vi "_TEST_ObjCacher.vi"() -> ()   [LabVIEW 2017]
uses:
  ObjectCacher-Operation.ctl
  a46cdb9f-ccaa-43c4-a046-aebf299bd719.vi
  e83d7f05-6254-462c-8cdd-b9405a50ceee.vi
  770d1e0a-3b1e-40e7-88fb-791e80b0e344.vi
  a343c373-1cd9-49a8-b7bb-35b9f087bed4.vi
  <vilib>/Utility/error.llb/Clear Errors.vi
  <userlib>/_OpenG.lib/md5/md5.llb/MD5 Message Digest (Hexadecimal String)__ogtk.vi
panel:
  out "names":string[](array[string])
  out "element 3":string
  out "data string 3":string
  out "element 2":string
  out "data string 2":string
  out "data string":string
  out "element":string
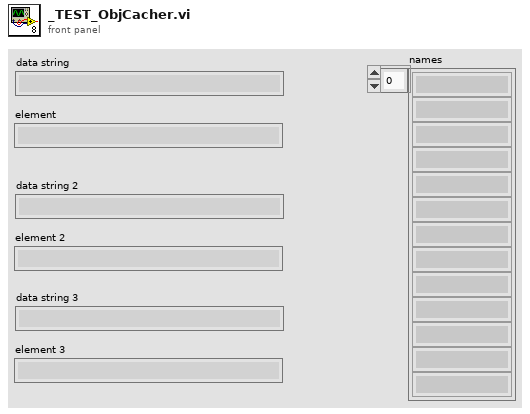
[diagram p1: front panel]
types:
  T1 = typedef "ObjectCacher-Operation.ctl" = enum16{"Reset", "Set", "Get", "Delete", "List", "<NONE>"}
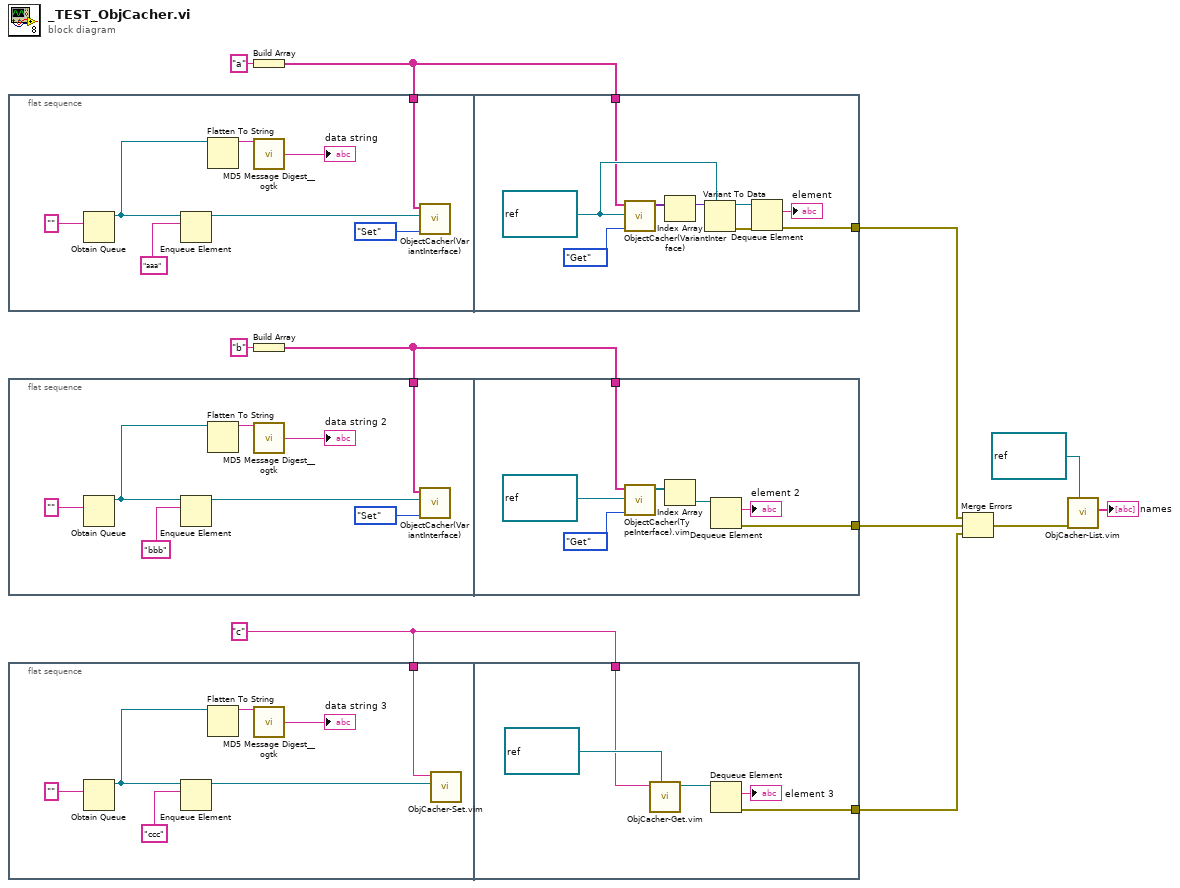
[diagram p0: block diagram]
diagram:
  w7 = "c" ("key")
  n1 = flat-sequence {
    tunnel: w10 -> [w12]
    tunnel: w10 -> [w24]
    tunnel: [w20] -> w4
    frame #0 {
      n2 = Obtain Queue(element data type="") -> (queue out=w16:refnum<queue>)  [unwired: 4 in, 2 out]
      n3 = Enqueue Element(queue=w16, element="aaa") -> (queue out=w18:refnum<queue>)  [unwired: 2 in, 2 out]
      n4 = Flatten To String(anything=w16) -> (data string=w15:string)  [unwired: 3 in, 2 out]
      n5 = call-poly <userlib>:"MD5 Message Digest__ogtk.vi"("Message"=w15) -> ("MD5 Message Digest"=→"data string":string)
      n6 = call "ObjectCacher(VariantInterface).vi"("Enum(Get)"=ObjectCacher-Operation."Set", "Variant"=w18, "key"=w12) -> ()  [unwired: 5 in, 4 out]
    }
    frame #1 {
      w28 = refnum<queue> refnum ("queue out")
      n7 = call "ObjectCacher(VariantInterface).vi"("Enum(Get)"=ObjectCacher-Operation."Get", "Variant"=w28, "key"=w24) -> ("values"=w22:variant[])  [unwired: 5 in, 3 out]
      n8 = Index Array(array=w22) -> (element=w21:variant)  [unwired: 1 in]
      n9 = Variant To Data(type=w28, Variant=w21) -> (data=w27:refnum<queue>, error out=w26:errorcluster)  [unwired: 1 in]
      n10 = Dequeue Element(queue=w27, error in (no error)=w26) -> (element=→"element":string, error out=w20:errorcluster)  [unwired: 1 in, 2 out]
    }
  }
  n11 = flat-sequence {
    tunnel: w9 -> [w29]
    tunnel: w9 -> [w41]
    tunnel: [w37] -> w6
    frame #0 {
      n12 = Obtain Queue(element data type="") -> (queue out=w33:refnum<queue>)  [unwired: 4 in, 2 out]
      n13 = Enqueue Element(queue=w33, element="bbb") -> (queue out=w35:refnum<queue>)  [unwired: 2 in, 2 out]
      n14 = Flatten To String(anything=w33) -> (data string=w32:string)  [unwired: 3 in, 2 out]
      n15 = call-poly <userlib>:"MD5 Message Digest__ogtk.vi"("Message"=w32) -> ("MD5 Message Digest"=→"data string 2":string)
      n16 = call "ObjectCacher(VariantInterface).vi"("Enum(Get)"=ObjectCacher-Operation."Set", "Variant"=w35, "key"=w29) -> ()  [unwired: 5 in, 4 out]
    }
    frame #1 {
      n17 = call "ObjectCacher(TypeInterface).vim"("Enum(Get)"=ObjectCacher-Operation."Get", "Variant"=refnum<queue> refnum ("queue out"), "key"=w41) -> ("values"=w39:refnum<queue>[])  [unwired: 5 in, 3 out]
      n18 = Index Array(array=w39) -> (element=w38:refnum<queue>)  [unwired: 1 in]
      n19 = Dequeue Element(queue=w38) -> (element=→"element 2":string, error out=w37:errorcluster)  [unwired: 2 in, 2 out]
    }
  }
  n20 = flat-sequence {
    tunnel: w7 -> [w44]
    tunnel: w7 -> [w52]
    tunnel: [w51] -> w3
    frame #0 {
      n21 = Obtain Queue(element data type="") -> (queue out=w48:refnum<queue>)  [unwired: 4 in, 2 out]
      n22 = Enqueue Element(queue=w48, element="ccc") -> (queue out=w45:refnum<queue>)  [unwired: 2 in, 2 out]
      n23 = Flatten To String(anything=w48) -> (data string=w47:string)  [unwired: 3 in, 2 out]
      n24 = call-poly <userlib>:"MD5 Message Digest__ogtk.vi"("Message"=w47) -> ("MD5 Message Digest"=→"data string 3":string)
      n25 = call "ObjCacher-Set.vim"("type"=w45, "Module Name"=w44) -> ()  [unwired: 7 in, 3 out]
    }
    frame #1 {
      n26 = call "ObjCacher-Get.vim"("type"=refnum<queue> refnum ("queue out"), "Module Name"=w52) -> ("Variant"=w53:refnum<queue>)  [unwired: 6 in, 3 out]
      n27 = Dequeue Element(queue=w53) -> (element=→"element 3":string, error out=w51:errorcluster)  [unwired: 2 in, 2 out]
    }
  }
  n28 = Build Array("a" ("key")) -> (w10:string[])
  n29 = Build Array("b" ("key")) -> (w9:string[])
  n30 = Merge Errors(w4, w6, w3) -> (w5:errorcluster)
  n31 = call "ObjCacher-List.vim"("type"=refnum<queue> refnum ("queue out"), "error in (no error)"=w5) -> ("names"=→"names":string[])  [unwired: 7 in, 2 out]
